vi "Lang Set Desc c.vi"(8 "error in (no error)":errorcluster, 10 "c":T1, 11 "LF2R IDE in":refnum<class "Main Panel.lvclass">) -> (0 "error out":errorcluster, 3 "LF2R IDE out":refnum<class "Main Panel.lvclass">)   [LabVIEW 2018, in "Framework.lvlib" / "Framework.lvclass"]
uses:
  Framework/Framework/Framework.lvclass
  Main Panel.lvclass
  D:/project/hobby/LabVIEW/LF2R/LabVIEW/Source/Actor/Framework/Framework/Framework.lvclass
  C:/Program Files (x86)/National Instruments/LabVIEW 2018/vi.lib/MGI/Panel Manager/Panel Actor/Panel Actor/Panel Actor.lvclass
  C:/Program Files (x86)/National Instruments/LabVIEW 2018/vi.lib/MGI/Monitored Actor/Monitored Actor/Monitored Actor/Monitored Actor.lvclass
  C:/Program Files (x86)/National Instruments/LabVIEW 2018/vi.lib/ActorFramework/Actor/Actor.lvclass
  Const Lang Property.ctl
  Const UI Desc Frame c.ctl
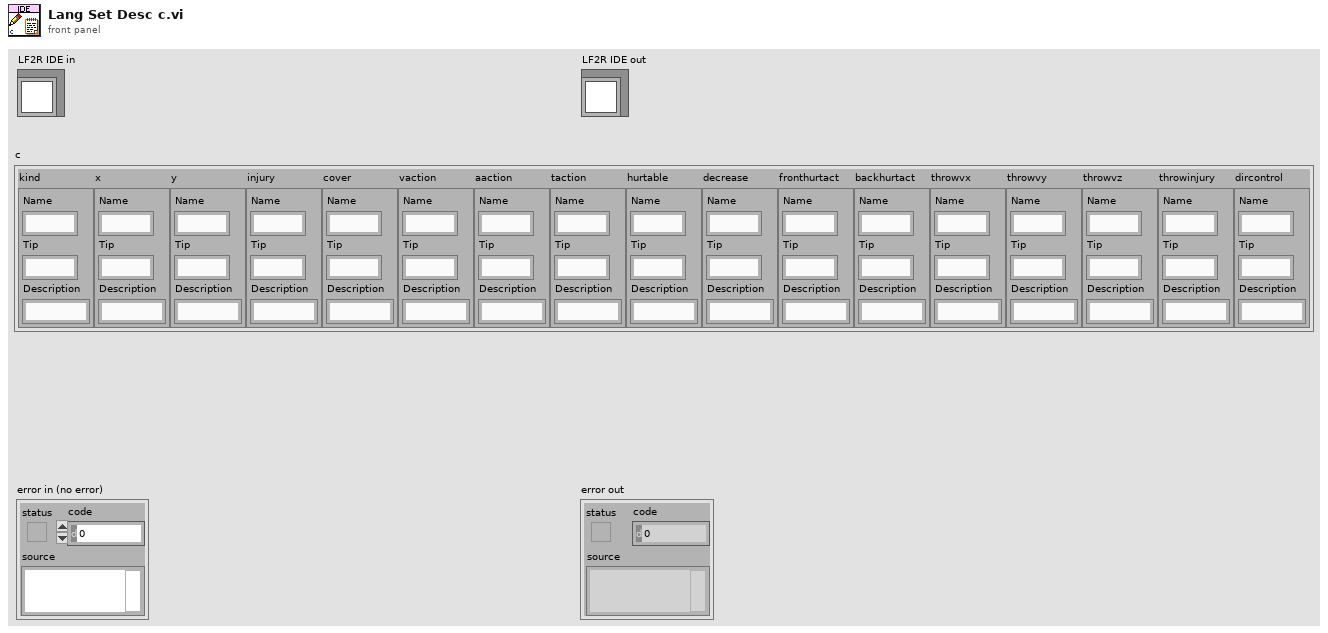
[diagram p1: front panel]
types:
  T1 = typedef "Framework.lvlib/Framework.lvclass/Const UI Desc Frame c.ctl" = cluster{"kind":T2, "x":T2, "y":T2, "injury":T2, "cover":T2, "vaction":T2, "aaction":T2, "taction":T2, "hurtable":T2, "decrease":T2, "fronthurtact":T2, "backhurtact":T2, "throwvx":T2, "throwvy":T2, "throwvz":T2, "throwinjury":T2, "dircontrol":T2}
  T2 = typedef "Framework.lvlib/Framework.lvclass/Const Lang Property.ctl" = cluster{"Name":string, "Tip":string, "Description":string}
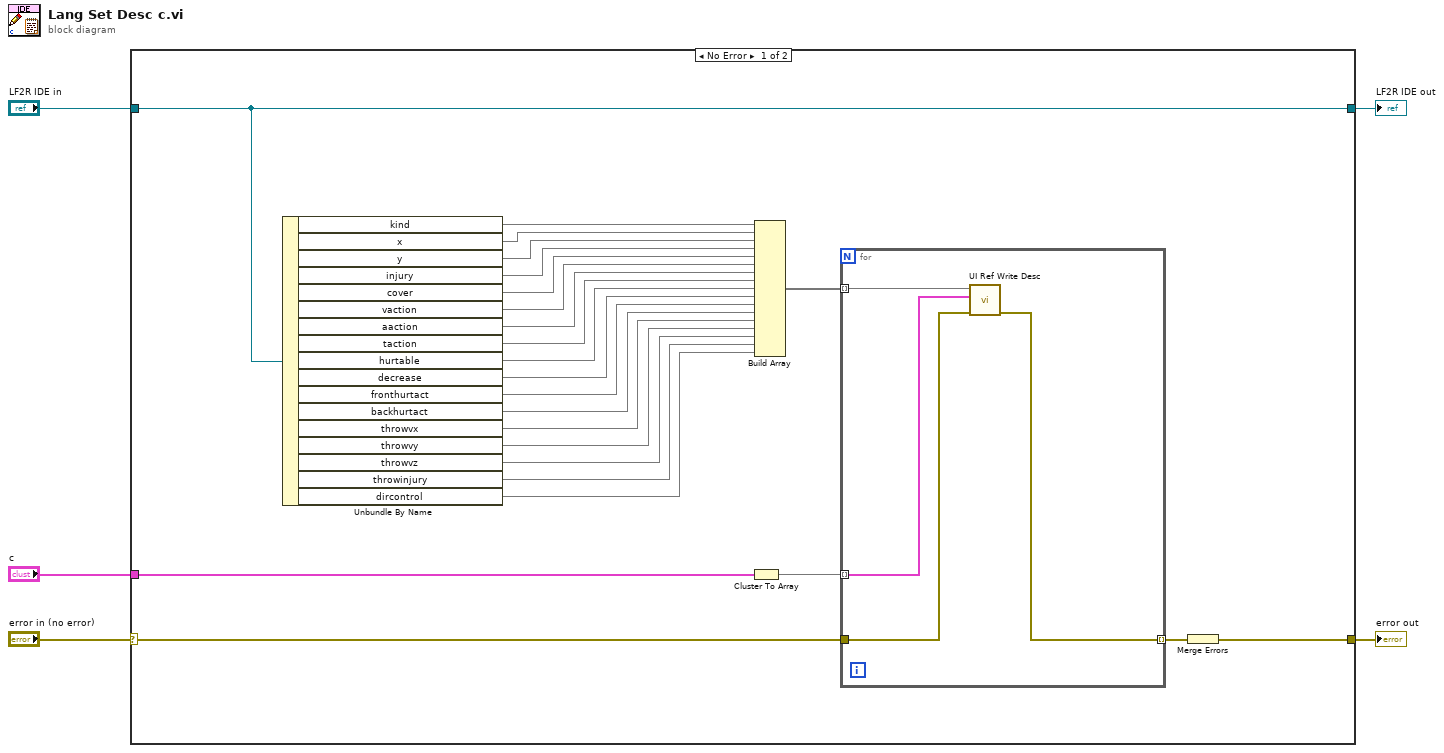
[diagram p0: block diagram]
diagram:
  n1 = case shown="No Error" "error in (no error)" {
    selector: "error in (no error)" -> [w25 w35]
    tunnel: [w23 w35] -> w4
    tunnel: [w29 w34] -> w2
    tunnel: "LF2R IDE in" -> [w29 w34]
    tunnel: "c" -> [w27 _]
    frame No Error {
      n2 = Unbundle By Name(w29) -> ("kind"=w22, "x"=w21, "y"=w20, "injury"=w19, "cover"=w18, "vaction"=w17, "aaction"=w16, "taction"=w15, "hurtable"=w14, "decrease"=w13, "fronthurtact"=w12, "backhurtact"=w11, "throwvx"=w10, "throwvy"=w9, "throwvz"=w8, "throwinjury"=w7, "dircontrol"=w6)
      n3 = Cluster To Array(cluster=w27) -> (array=w26:T2[])
      n4 = Build Array(w22, w21, w20, w19, w18, w17, w16, w15, w14, w13, w12, w11, w10, w9, w8, w7, w6) -> (w28:void[])
      n5 = for {
        tunnel: w28 -> [w30] mode=indexing
        tunnel: w26 -> [w33] mode=indexing
        tunnel: w25 -> [w32]
        tunnel: [w31] -> w24 mode=indexing
        n6 = call "UI Ref Write Desc.vi"("error in (no error)"=w32, "UI Property"=w33, "UI Ref"=w30) -> ("error out"=w31:errorcluster)  [unwired: 8 in]
      }
      n7 = Merge Errors(w24) -> (w23:errorcluster)
    }
    frame Error {
    }
  }
  "error out" <- w4
  "LF2R IDE out" <- w2
